vi "Create Message Getter (from Accessor).vi"(8 "error in (no error)":errorcluster, 10 "RPC Message Name":string, 11 "RPC Messages Folder (ProjectItem) in":refnum<vi>) -> (0 "error out":errorcluster, 1 "Created ?":bool, 2 "Getter VI out":refnum<vi>, 3 "RPC Messages Folder (ProjectItem) out":refnum<vi>)   [LabVIEW 2019, in "gRPC Template Creation Utility.lvlib"]
uses:
  gRPC Template Creation Utility.lvlib
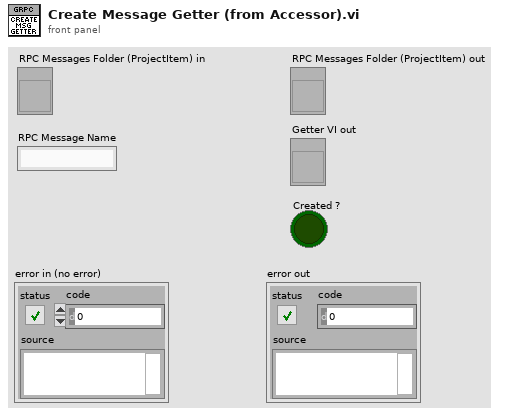
[diagram p1: front panel]
types:
  T1 = enum32{"invalid VI type", "Standard VI", "Control VI", "Global VI", "Polymorphic VI", "Configuration VI", "SubSystem", "Facade VI", "Method VI"}
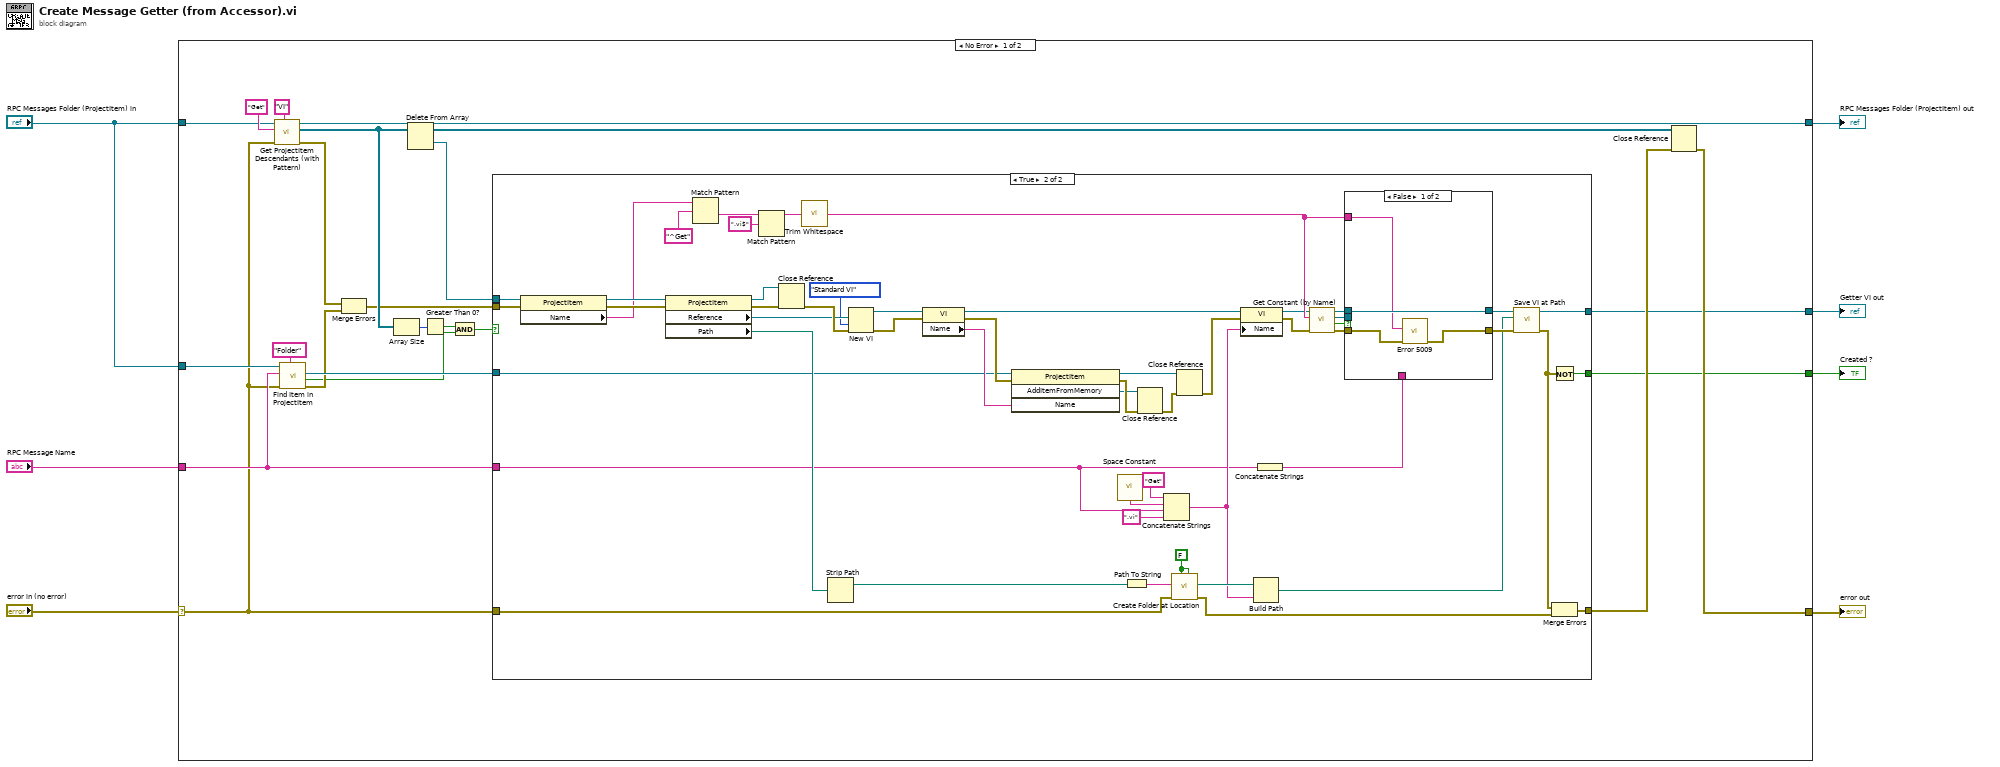
[diagram p0: block diagram]
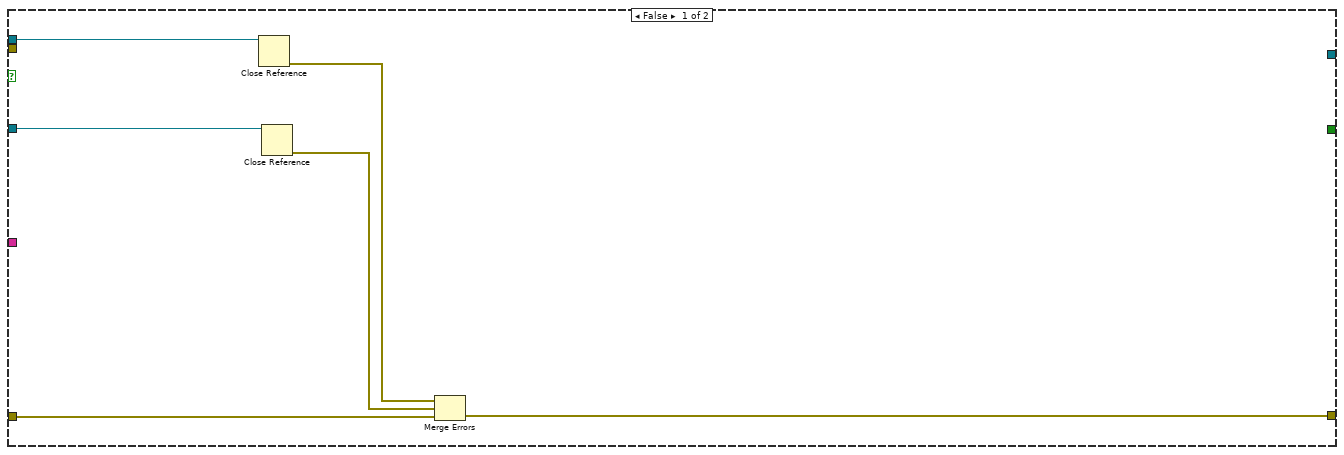
[diagram p2: hidden frame]
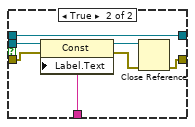
[diagram p3: hidden frame]
diagram:
  n1 = case shown="No Error" "error in (no error)" {
    selector: "error in (no error)" -> [w13 w101]
    tunnel: "RPC Message Name" -> [w25 _]
    tunnel: "RPC Messages Folder (ProjectItem) in" -> [w23 _]
    tunnel: "RPC Messages Folder (ProjectItem) in" -> [w18 w100]
    tunnel: [w11 w101] -> w4
    tunnel: [w10 w100] -> w3
    tunnel: [w9 _] -> w2
    tunnel: [w8 _] -> w1
    frame No Error {
      n2 = call "Get ProjectItem Descendants (with Pattern).vi"("Type"="VI", "error in (no error)"=w13, "Pattern"="Get", "ProjectItem in"=w18) -> ("error out"=w17:errorcluster, "ProjectItem descendents"=w24:refnum<vi>[], "ProjectItem out"=w10:refnum<vi>)  [unwired: 5 in]
      n3 = call "Find Item in ProjectItem.vi"("Item Type"="Folder", "error in (no error)"=w13, "Name"=w25, "ProjectItem in"=w23) -> ("error out"=w16:errorcluster, "Found ?"=w15:bool, "Item Refnum out"=w21:refnum<vi>)  [unwired: 4 in, 1 out]
      n4 = Merge Errors(w17, w16) -> (w14:errorcluster)
      n5 = Array Size(array=w24) -> (size(s)=w22:i32)
      n6 = Delete From Array(array=w24) -> (deleted portion=w27:refnum<vi>, array with subset deleted=w30:refnum<vi>[])  [unwired: 2 in]
      n7 = Greater Than 0?(x=w22) -> (x > 0?=w20:bool)
      n8 = And(x=w20, y=w15) -> (x .and. y?=w19:bool)
      n9 = case shown="True" w19 {
        tunnel: w25 -> [_ w48]
        tunnel: [w33 w85] -> w12
        tunnel: [_ w44] -> w8
        tunnel: w27 -> [w36 w60]
        tunnel: [_ w70] -> w9
        tunnel: w21 -> [w31 w65]
        tunnel: w13 -> [w32 w64]
        tunnel: w14 -> [_ w59]
        frame False {
          n10 = Close Reference(reference=w36) -> (error out=w34:errorcluster)  [unwired: 1 in]
          n11 = Close Reference(reference=w31) -> (error out=w35:errorcluster)  [unwired: 1 in]
          n12 = Merge Errors(w34, w35, w32) -> (w33:errorcluster)
        }
        frame True {
          w83 = FALSE ("Use Relative (F)")
          n13 = property class="ProjectItem"(reference=w60, error in=w59) -> (reference out=w58:refnum<vi>, error out=w57:errorcluster, "Name"=w56:string)
          n14 = property class="ProjectItem"(reference=w58, error in=w57) -> (reference out=w88:refnum<vi>, error out=w86:errorcluster, "Reference"=w76:refnum<vi>, "Path"=w79:path)
          n15 = Match Pattern(string=w56, regular expression="^Get") -> (after substring=w54:string)  [unwired: 1 in, 3 out]
          n16 = Match Pattern(string=w54, regular expression=".vi$") -> (before substring=w41:string)  [unwired: 1 in, 3 out]
          n17 = Close Reference(reference=w88, error in (no error)=w86) -> (error out=w87:errorcluster)
          n18 = call <vilib>:"Trim Whitespace.vi"("string"=w41) -> ("trimmed string"=w52:string)  [unwired: 1 in]
          n19 = Strip Path(path=w79) -> (stripped path=w37:path)  [unwired: 1 out]
          n20 = New VI(8:w87, 9:T1."Standard VI" ("vi type (standard vi)"), 10:w76) -> (0:w75:errorcluster, 3:w73:refnum<vi>)  [unwired: 1 in, 3 out]
          n21 = property class="VI"(reference=w73, error in=w75) -> (reference out=w80:refnum<vi>, error out=w81:errorcluster, "Name"=w77:string)
          n22 = invoke class="ProjectItem" method="AddItemFromMemory"(reference=w65, error in=w81, "Name"=w77) -> (reference out=w72:refnum<vi>, error out=w63:errorcluster, "AddItemFromMemory"=w62:refnum<vi>)  [unwired: 1 in, 1 out]
          n23 = call <vilib>:"Space Constant.vi"() -> ("String"=w68:string)
          n24 = Path To String(path=w37) -> (string=w78:string)
          n25 = Close Reference(reference=w62, error in (no error)=w63) -> (error out=w61:errorcluster)
          n26 = Concatenate Strings("Get" ("string"), w68, w48, ".vi" ("string")) -> (w66:string)
          n27 = call "Create Folder at Location.vi"("Override existing (F)"=w83, "Use Relative (F)"=w83, "Error In"=w64, "Path"=w78) -> ("Error Out"=w84:errorcluster, "Full path out"=w82:path)  [unwired: 5 in, 1 out]
          n28 = Close Reference(reference=w72, error in (no error)=w61) -> (error out=w71:errorcluster)
          n29 = property class="VI"(reference=w80, error in=w71, "Name"=w66) -> (reference out=w50:refnum<vi>, error out=w49:errorcluster)
          n30 = Build Path(base path=w82, name or relative path=w66) -> (appended path=w43:path)
          n31 = Concatenate Strings(w48) -> (w47:string)
          n32 = call "Get Constant (by Name).vi"("error in (no error)"=w49, "Constant Label"=w52, "Owner VI in"=w50) -> ("error out"=w46:errorcluster, "Found ?"=w40:bool, "Const ref out"=w51:refnum<vi>, "Owner VI out"=w39:refnum<vi>)  [unwired: 5 in]
          n33 = case shown="False" w40 {
            tunnel: w51 -> [_ w99]
            tunnel: w47 -> [_ w98]
            tunnel: w46 -> [w91 w97]
            tunnel: [w90 w94] -> w45
            tunnel: w39 -> [w92 w93]
            tunnel: [w92 w93] -> w38
            tunnel: w52 -> [w89 _]
            frame False {
              n34 = call "Error 5009.vi"("error in (no error)"=w91, "Cluster Definition Constant"=w89) -> ("error out"=w90:errorcluster)  [unwired: 9 in]
            }
            frame True {
              n35 = property class="Const"(reference=w99, error in=w97, "Label.Text"=w98) -> (reference out=w96:refnum<vi>, error out=w95:errorcluster)
              n36 = Close Reference(reference=w96, error in (no error)=w95) -> (error out=w94:errorcluster)
            }
          }
          n37 = call "Save VI at Path.vi"("error in (no error)"=w45, "Path"=w43, "VI in"=w38) -> ("error out"=w42:errorcluster, "VI out"=w44:refnum<vi>)  [unwired: 6 in, 1 out]
          n38 = Not(x=w42) -> (.not. x?=w70:bool)
          n39 = Merge Errors(w42, w84) -> (w85:errorcluster)
        }
      }
      n40 = Close Reference(reference=w30, error in (no error)=w12) -> (error out=w11:errorcluster)
    }
    frame Error {
    }
  }
  "error out" <- w4
  "RPC Messages Folder (ProjectItem) out" <- w3
  "Created ?" <- w2
  "Getter VI out" <- w1
